vi "(auto) Recover def pos (SubVI).vi"(4 "Right Encoder Ref In 2":T1, 6 "Left Encoder Ref In":T1, 8 "error in (no error)":errorcluster, 9 "CurDot":T7(ring), 10 "Left_enc":i32[](array[numeric]), 11 "Right_enc":i32[](array[numeric])) -> (0 "error out":errorcluster, 3 "Recovered":bool)   [LabVIEW 2017]
uses:
  <vilib>/myRIO/Instrument Drivers/Onboard IO/Encoder/typedefs/Encoder Reference.ctl
  <vilib>/myRIO/Common/Instrument Driver Framework/Utilities/typedefs/myRIO Generic Hardware Reference.ctl
  <vilib>/myRIO/Common/Instrument Driver Framework/Utilities/typedefs/Hardware Version Enum.ctl
  <vilib>/myRIO/Common/Instrument Driver Framework/Utilities/typedefs/myRIO v1.0 Reference.ctl
  <vilib>/myRIO/Common/Instrument Driver Framework/Utilities/typedefs/Generic FPGA Reference.ctl
  <vilib>/myRIO/Common/Instrument Driver Framework/myRIO v1.0/Encoder/typedefs/Encoder Channels Enum.ctl
  <vilib>/myRIO/Instrument Drivers/Onboard IO/DIO/typedefs/DIO Reference.ctl
  <vilib>/myRIO/Common/Instrument Driver Framework/myRIO v1.0/DIO/typedefs/DIO Channels List.ctl
  <vilib>/myRIO/Common/Instrument Driver Framework/myRIO v1.0/DIO/typedefs/DIO Channels Enum.ctl
  <vilib>/userdefined/High Color/nirio_resource_hc.ctl
  <vilib>/myRIO/Common/Instrument Driver Framework/Utilities/vis/Is FPGA Ref Available.vi
  <vilib>/myRIO/Common/Instrument Driver Framework/myRIO v1.0/DIO/vis/myRIO v1.1 Open DIO.vi
  <vilib>/myRIO/Instrument Drivers/Onboard IO/DIO/vis/Write.vi
  <vilib>/myRIO/Common/Instrument Driver Framework/Utilities/vis/Validate Channels.vi
  <vilib>/myRIO/Common/Instrument Driver Framework/myRIO v1.0/DIO/vis/myRIO v1.0 Reserve DIO.vi
  <vilib>/myRIO/Common/Instrument Driver Framework/myRIO v1.0/Resource Manager/vis/myRIO v1.0 Reserve Channel List.vi
  <vilib>/myRIO/Common/Instrument Driver Framework/myRIO v1.0/DIO/vis/myRIO v1.0 Build MUX Configuration DIO.vi
  <vilib>/myRIO/Common/Instrument Driver Framework/myRIO v1.0/Resource Manager/vis/myRIO v1.0 Reserve Channel.vi
  <vilib>/myRIO/Common/Instrument Driver Framework/myRIO v1.0/Resource Manager/vis/myRIO v1.0 Unreserve Channel.vi
  <vilib>/myRIO/Common/Instrument Driver Framework/myRIO v1.0/Resource Manager/vis/myRIO v1.0 Create Configuration List.vi
  <vilib>/myRIO/Common/Instrument Driver Framework/myRIO v1.0/Resource Manager/vis/myRIO v1.0 Build Mutex Name.vi
  <vilib>/Utility/error.llb/Error Cluster From Error Code.vi
  <vilib>/myRIO/Common/Instrument Driver Framework/myRIO v1.0/Encoder/vis/myRIO v1.0 Read Encoder.vi
  <vilib>/Utility/VariantDataType/GetNumericInfo.vi
  <vilib>/myRIO/Common/Instrument Driver Framework/myRIO v1.0/myRIO v1.1 Open.vi
  <vilib>/myRIO/Common/Instrument Driver Framework/Utilities/vis/IO Manager.vi
  <vilib>/myRIO/Common/Instrument Driver Framework/Utilities/vis/Configuration Manager.vi
  <vilib>/myRIO/Common/Instrument Driver Framework/myRIO v1.0/Resource Manager/vis/myRIO v1.0 Configure IO.vi
  <vilib>/myRIO/Common/Instrument Driver Framework/myRIO v1.0/myRIO v1.0 Close.vi
  <vilib>/myRIO/Common/Instrument Driver Framework/myRIO v1.0/DIO/vis/myRIO v1.0 Write DIO.vi
  <vilib>/myRIO/Express VI/Onboard IO/DO/DO Express VI.xnode
  <vilib>/myRIO/Instrument Drivers/Onboard IO/DIO/vis/myRIO DIO Open.xnode
  <vilib>/myRIO/Instrument Drivers/Onboard IO/Encoder/Encoder.lvlib
  <vilib>/myRIO/Instrument Drivers/Onboard IO/DIO/DIO.lvlib
panel:
  in  "Stop Button":bool
  in  "Range":i32
  out "need R_enc":i32
  out "need L_enc":i32
  out "cur L_enc":i32
  out "cur R_enc":i32
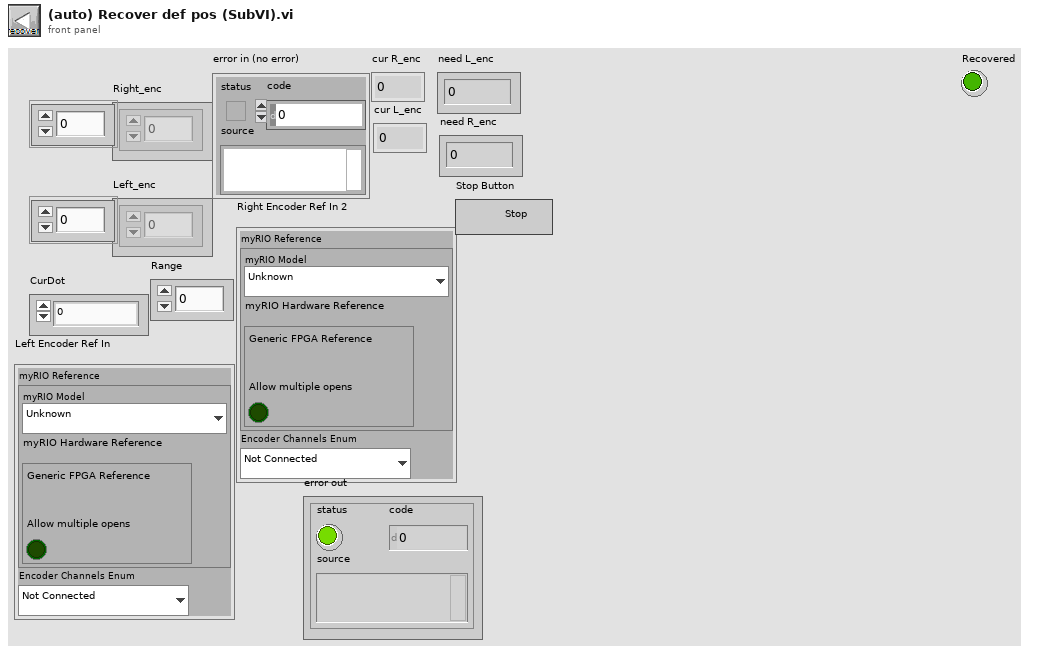
[diagram p1: front panel]
types:
  T1 = typedef "Encoder.lvlib/Encoder Reference.ctl" = cluster{"myRIO Reference":T2, "Encoder Channels Enum":T6}
  T2 = typedef "myRIO Generic Hardware Reference.ctl" = cluster{"myRIO Model":T3, "myRIO Hardware Reference":T4}
  T3 = typedef "Hardware Version Enum.ctl" = enum16{"Unknown", "myRIO-1900", "myRIO-1950", "roboRIO", "NI ELVIS RIO CM"}
  T4 = typedef "myRIO v1.0 Reference.ctl" = cluster{"Generic FPGA Reference":T5, "Allow multiple opens":bool}
  T5 = typedef "Generic FPGA Reference.ctl" = refnum<k20>
  T6 = typedef "Encoder Channels Enum.ctl" = enum16{"Not Connected", "C/ENC0", "C/ENC1", "A/ENC", "B/ENC", "DIO/ENC0", "DIO/ENC1", "DIO/ENC2", "DIO/ENC3", "DIO/ENC4"}
  T7 = enum16{"0", "1", "2", "3", "4", "5", "6", "7", "8", "9", "10", "11", "12", "13", "14", "15", "16", "17", "18", "19", "20", "21", "22", "23", "24", "25", "26", "27", "28", "29", "30", "31", "32", "33", "34", "35"}
  T8 = typedef "DIO.lvlib/DIO Reference.ctl" = cluster{"myRIO Reference":T2, "DIO Channels List":T9}
  T9 = typedef "DIO Channels List.ctl" = T10[]
  T10 = typedef "DIO Channels Enum.ctl" = enum16{"Not Connected", "C/DIO0", "C/DIO1", "C/DIO2", "C/DIO3", "C/DIO4", "C/DIO5", "C/DIO6", "C/DIO7", "A/DIO0", "A/DIO1", "A/DIO2", "A/DIO3", "A/DIO4", "A/DIO5", "A/DIO6", "A/DIO7", "A/DIO8", "A/DIO9", "A/DIO10", "A/DIO11", "A/DIO12", "A/DIO13", "A/DIO14", "A/DIO15", "B/DIO0", "B/DIO1", "B/DIO2", "B/DIO3", "B/DIO4", "B/DIO5", "B/DIO6", "B/DIO7", "B/DIO8", "B/DIO9", "B/DIO10", "B/DIO11", "B/DIO12", "B/DIO13", "B/DIO14", "B/DIO15", "LED0", "LED1", "LED2", "LED3", "Button0", "DIO/DIO0", "DIO/DIO1", "DIO/DIO2", "DIO/DIO3", "DIO/DIO4", "DIO/DIO5", "DIO/DIO6", "DIO/DIO7", "DIO/DIO8", "DIO/DIO9", "SPI/CS0", "SPI/CS1", "SPI/CS2", "SPI/CS3", "LED RADIO (Green)", "LED RADIO (Red)", "LED COMM (Green)", "LED COMM (Red)", "LED MODE (Green)", "LED MODE (Red)"}
  T11 = typedef "nirio_resource_hc.ctl" = tag
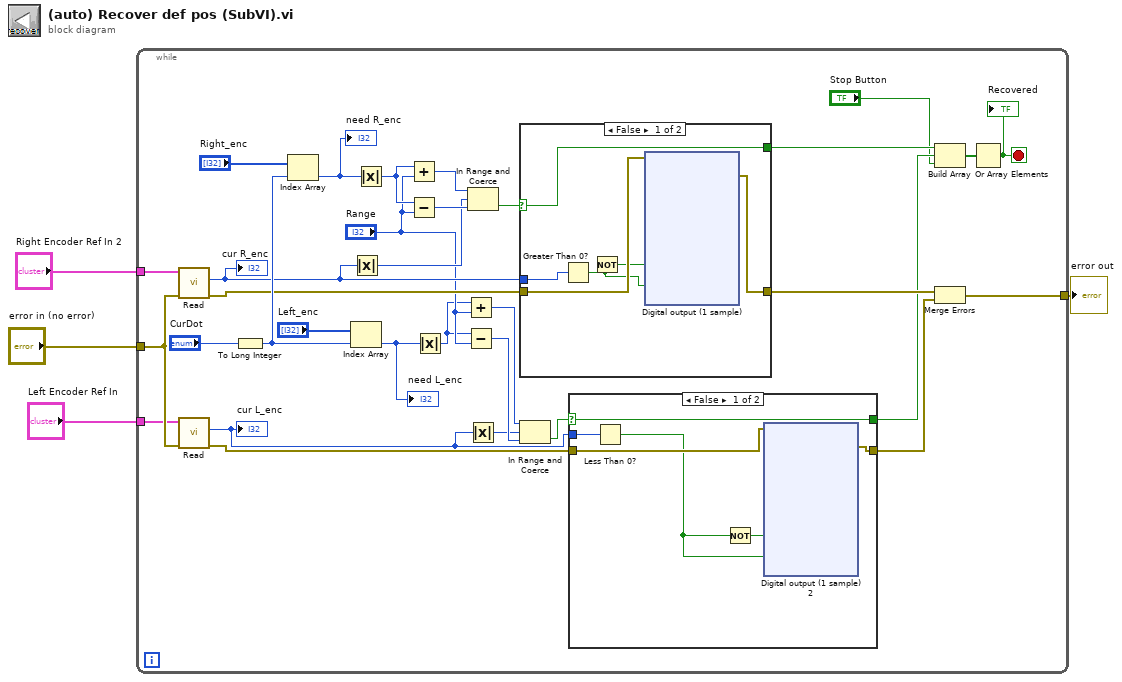
[diagram p0: block diagram]
diagram:
  n1 = while {
    tunnel: "error in (no error)" -> [w36]
    tunnel: "Left Encoder Ref In" -> [w35]
    tunnel: "Right Encoder Ref In 2" -> [w34]
    tunnel: [w14] -> w1
    stop <- w12 stop-if-true
    n2 = call <vilib>:"Read.vi"("error in (no error)"=w36, "Encoder Ref In"=w34) -> ("error out"=w17:errorcluster, "Counter Value"=w19:i32)  [unwired: 5 in, 3 out]
    "cur R_enc" <- w19
    n3 = call <vilib>:"Read.vi"("error in (no error)"=w36, "Encoder Ref In"=w35) -> ("error out"=w16:errorcluster, "Counter Value"=w18:i32)  [unwired: 5 in, 3 out]
    "cur L_enc" <- w18
    n4 = To Long Integer(number="CurDot") -> (32bit integer=w30:i32)
    n5 = Index Array(array="Right_enc", index=w30) -> (element=w25:i32)
    "need R_enc" <- w25
    n6 = Index Array(array="Left_enc", index=w30) -> (element=w27:i32)
    "need L_enc" <- w27
    n7 = Absolute Value(x=w19) -> (abs(x)=w20:i32)
    n8 = Absolute Value(x=w25) -> (abs(x)=w7:i32)
    n9 = Add(x=w7, y="Range") -> (x+y=w24:i32)
    n10 = Subtract(x=w7, y="Range") -> (x-y=w23:i32)
    n11 = Absolute Value(x=w27) -> (abs(x)=w5:i32)
    n12 = Add(x=w5, y="Range") -> (x+y=w26:i32)
    n13 = Subtract(x=w5, y="Range") -> (x-y=w22:i32)
    n14 = In Range and Coerce(upper limit=w24, x=w20, lower limit=w23) -> (In Range?=w28:bool)  [unwired: 1 out]
    n15 = Absolute Value(x=w18) -> (abs(x)=w21:i32)
    n16 = case shown="False" w28 {
      selector: w28 -> [w83 w123]
      tunnel: w19 -> [w86 _]
      tunnel: w17 -> [w85 w124]
      tunnel: [w84 w124] -> w13
      tunnel: [w83 w123] -> w10
      frame False {
        n17 = Greater Than 0?(x=w86) -> (x > 0?=w82:bool)
        n18 = Not(x=w82) -> (.not. x?=w81:bool)
        n19 = xnode "Digital output (1 sample)"("Right+ (A/DIO7 (Pin 25))"=w81, "Right- (A/DIO13 (Pin 26))"=w82, "error in (no error)"=w85) -> ("error out"=w84:errorcluster)
      }
      frame True {
      }
    }
    n20 = In Range and Coerce(upper limit=w26, x=w21, lower limit=w22) -> (In Range?=w29:bool)  [unwired: 1 out]
    n21 = case shown="False" w29 {
      selector: w29 -> [w38 w79]
      tunnel: w18 -> [w41 _]
      tunnel: w16 -> [w40 w80]
      tunnel: [w39 w80] -> w15
      tunnel: [w38 w79] -> w9
      frame False {
        n22 = Less Than 0?(x=w41) -> (x < 0?=w37:bool)
        n23 = Not(x=w37) -> (.not. x?=w42:bool)
        n24 = xnode "Digital output (1 sample) 2"("Left+ (A/DIO5 (Pin 21))"=w42, "Left- (A/DIO6 (Pin 23))"=w37, "error in (no error)"=w40) -> ("error out"=w39:errorcluster)
      }
      frame True {
      }
    }
    n25 = Build Array(w10, w9, "Stop Button") -> (w11:bool[])
    n26 = Merge Errors(w13, w15) -> (w14:errorcluster)
    n27 = Or Array Elements(Boolean array=w11) -> (logical OR=w12:bool)
    "Recovered" <- w12
  }
  "error out" <- w1
